vi "fill in_static.vi"   [LabVIEW 2023]
types:
  T1 = enum16{"Initialize", "Absolute Position", "Relative Pickup", "Relative Dispense", "Swich valve", "Bypass"}
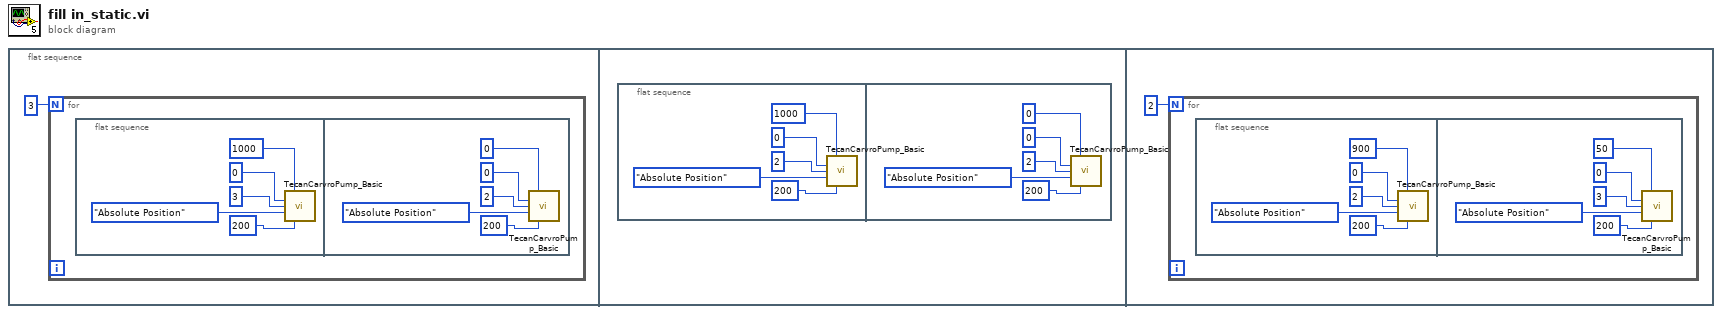
[diagram p0: block diagram]
diagram:
  n1 = flat-sequence {
    frame #0 {
      n2 = for {
        N: 3 -> [_]
        n3 = flat-sequence {
          frame #0 {
            n4 = call "TecanCarvroPump_Basic.vi"("Volume (μL)"=u16 1000, "TecanPump address"=u8 0, "Valve"=u8 3, "Mode"=T1."Absolute Position", "Speed (μL/s)"=u16 200) -> ()  [unwired: 10 in, 1 out]
          }
          frame #1 {
            n5 = call "TecanCarvroPump_Basic.vi"("Volume (μL)"=u16 0, "TecanPump address"=u8 0, "Valve"=u8 2, "Mode"=T1."Absolute Position", "Speed (μL/s)"=u16 200) -> ()  [unwired: 10 in, 1 out]
          }
        }
      }
    }
    frame #1 {
      n6 = flat-sequence {
        frame #0 {
          n7 = call "TecanCarvroPump_Basic.vi"("Volume (μL)"=u16 1000, "TecanPump address"=u8 0, "Valve"=u8 2, "Mode"=T1."Absolute Position", "Speed (μL/s)"=u16 200) -> ()  [unwired: 10 in, 1 out]
        }
        frame #1 {
          n8 = call "TecanCarvroPump_Basic.vi"("Volume (μL)"=u16 0, "TecanPump address"=u8 0, "Valve"=u8 2, "Mode"=T1."Absolute Position", "Speed (μL/s)"=u16 200) -> ()  [unwired: 10 in, 1 out]
        }
      }
    }
    frame #2 {
      n9 = for {
        N: 2 -> [_]
        n10 = flat-sequence {
          frame #0 {
            n11 = call "TecanCarvroPump_Basic.vi"("Volume (μL)"=u16 900, "TecanPump address"=u8 0, "Valve"=u8 2, "Mode"=T1."Absolute Position", "Speed (μL/s)"=u16 200) -> ()  [unwired: 10 in, 1 out]
          }
          frame #1 {
            n12 = call "TecanCarvroPump_Basic.vi"("Volume (μL)"=u16 50, "TecanPump address"=u8 0, "Valve"=u8 3, "Mode"=T1."Absolute Position", "Speed (μL/s)"=u16 200) -> ()  [unwired: 10 in, 1 out]
          }
        }
      }
    }
  }
